vi "DIAdem String Variable Get.vi"(8 "error in (no error)":errorcluster, 10 "Variable Name":string, 11 "DIAdem Reference":T1) -> (0 "error out":errorcluster, 2 "Value":string, 3 "DIAdem Reference":T1)   [LabVIEW 2017]
doc: "Read specified string variable from DIAdem."
uses:
  <vilib>/ExportToExcel/DIAdem Reference.ctl
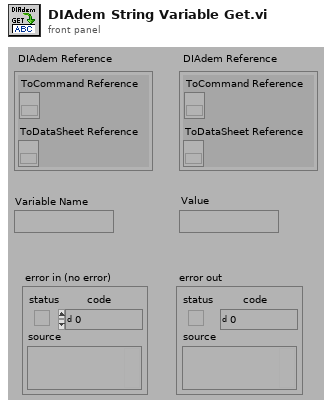
[diagram p1: front panel]
types:
  T1 = typedef "DIAdem Reference.ctl" = cluster{"ToCommand Reference":refnum<k7>, "ToDataSheet Reference":refnum<k7>}
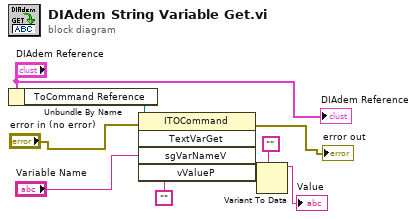
[diagram p0: block diagram]
diagram:
  n1 = Unbundle By Name("DIAdem Reference") -> ("ToCommand Reference"=w4:refnum<k7>)
  n2 = invoke class="ITOCommand" method="TextVarGet"(reference=w4, error in="error in (no error)", "sgVarNameV"="Variable Name", "vValueP"="") -> (error out=→"error out":errorcluster, "vValueP"=w8:variant)  [unwired: 1 in, 3 out]
  n3 = Variant To Data(type="", Variant=w8) -> (data=→"Value":string)  [unwired: 1 in, 1 out]
  "DIAdem Reference" <- "DIAdem Reference"
